vi "Disabled.vi"(7 "Robot Mode":T2, 10 "Match Info":T1={"Autonomous Elapsed Seconds"=0.0, "TeleOp Elapsed Seconds"=0.0, "Disabled Elapsed Seconds"=0.0, "Visited Autonomous"=FALSE, "Visited TeleOp"=FALSE, "Visited Disabled"=FALSE, "Autonomous Settings"={"Autonomous Style"=enum."Independent", "VI Refnum"=refnum}}, 11 "Call Context":T3) -> ()   [LabVIEW 2012]
doc: "This VI is called each time a disabled packet is received from the DS. It is often used to prepare for the next robot mode, to calibrate sensors, etc."
uses:
  <vilib>/Rock Robotics/WPI/DriverStation/WPI_DriverStationDerivedRobotMode.ctl
  <vilib>/Rock Robotics/WPI/DriverStation/WPI_DriverStationRobotMode2.ctl
  <vilib>/Rock Robotics/WPI/DriverStation/WPI_DriverStationMatch Info.ctl
  Robot Global Data.vi
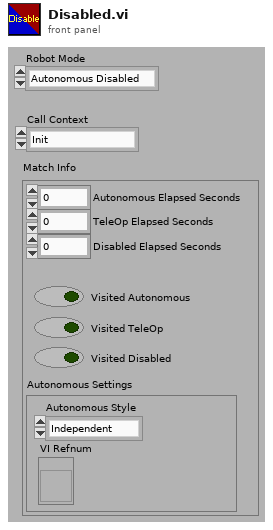
[diagram p1: front panel]
types:
  T1 = typedef "WPI_DriverStationMatch Info.ctl" = cluster{"Autonomous Elapsed Seconds":dbl, "TeleOp Elapsed Seconds":dbl, "Disabled Elapsed Seconds":dbl, "Visited Autonomous":bool, "Visited TeleOp":bool, "Visited Disabled":bool, "Autonomous Settings":cluster{"Autonomous Style":enum16{"Iterative", "Independent"}, "VI Refnum":refnum<vi>}}
  T2 = typedef "WPI_DriverStationRobotMode2.ctl" = enum16{"Autonomous Disabled", "Autonomous Enabled", "Teleop Disabled", "Teleop Enabled", "Timeout", "Finish", "Test Disabled", "Test Enabled"}
  T3 = typedef "WPI_DriverStationDerivedRobotMode.ctl" = enum16{"Init", "Execute", "Stop"}
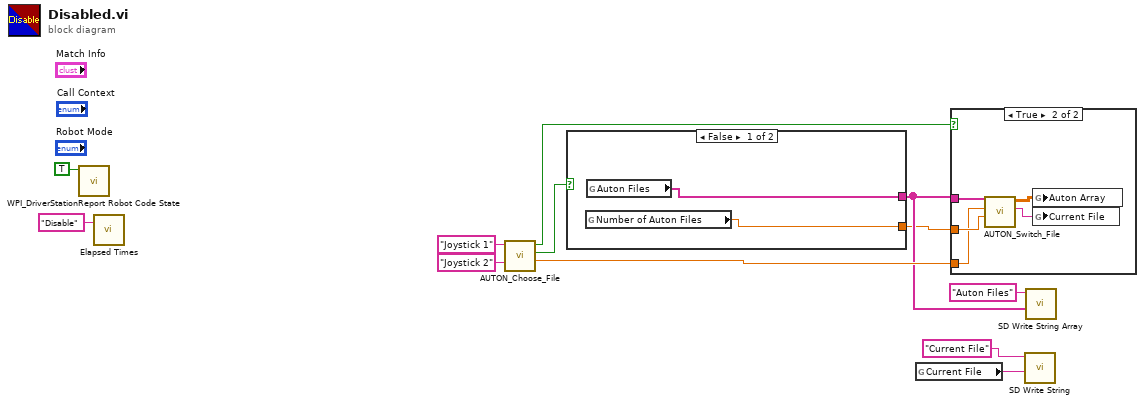
[diagram p0: block diagram]
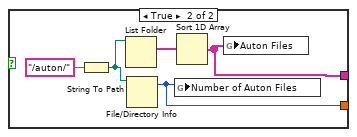
[diagram p3: hidden frame]
diagram:
  n1 = call <vilib>:"WPI_DriverStationReport Robot Code State.vi"("Disabled"=TRUE ("Autonomous")) -> ()  [unwired: 10 in, 1 out]
  n2 = call "Elapsed Times.vi"("Call Name"="Disable") -> ()  [unwired: 2 in, 1 out]
  n3 = call "AUTON_Choose_File.vi"("Joystick 2 Refnum"="Joystick 2", "Joystick 1 Refnum"="Joystick 1") -> ("Auton File"=w9:dbl, "Refresh"=w8:bool, "Allow Change"=w7:bool)  [unwired: 7 in]
  n4 = case shown="False" w8 {
    tunnel: [w13 w16] -> w4
    tunnel: [w14 w15] -> w6
    frame False {
      n5 = global read "Robot Global Data.vi" "Number of Auton Files"() -> (w13:dbl)
      n6 = global read "Robot Global Data.vi" "Auton Files"() -> (w14:string[])
    }
    frame True {
      n7 = String To Path(string="/auton/") -> (path=w18:path)
      n8 = List Folder(path=w18) -> (filenames=w17:string[])  [unwired: 3 in, 3 out]
      n9 = File/Directory Info(path=w18) -> (size=w16:i64)  [unwired: 1 in, 6 out]
      n10 = global write "Robot Global Data.vi" "Number of Auton Files"(w16) -> ()
      n11 = Sort 1D Array(array=w17) -> (sorted array=w15:string[])
      n12 = global write "Robot Global Data.vi" "Auton Files"(w15) -> ()
    }
  }
  n13 = global read "Robot Global Data.vi" "Current File"() -> (w3:string)
  n14 = case shown="True" w7 {
    tunnel: w9 -> [_ w22]
    tunnel: w6 -> [_ w24]
    tunnel: w4 -> [_ w23]
    frame False {
    }
    frame True {
      n15 = call "AUTON_Switch_File.vi"("Number of Auton Files"=w23, "Auton File"=w22, "Auton Files"=w24) -> ("Current File"=w21:string, "Auton Array"=w20:dbl[][])  [unwired: 7 in]
      n16 = global write "Robot Global Data.vi" "Auton Array"(w20) -> ()
      n17 = global write "Robot Global Data.vi" "Current File"(w21) -> ()
    }
  }
  n18 = call <vilib>:"SD Write String.vi"("String"=w3, "Name"="Current File") -> ()  [unwired: 8 in, 2 out]
  n19 = call <vilib>:"SD Write String Array.vi"("String Array"=w6, "Name"="Auton Files") -> ()  [unwired: 8 in, 2 out]
